vi "Test.vi"   [LabVIEW 2018, in "Scripts.lvlib"]
uses:
  Scripts.lvlib
  <vilib>/addons/_JKI Toolkits/Caraya/classes/Test/Test.lvclass
  tests/Toolkit/Toolkit.lvlib
  <vilib>/Field R&D Services/Labricator/Toolkit/Labricator.lvlib
panel:
  # "Overview: Runs all of tests this project\nRequirements: LabVIEW, Caraya Unit Test Framework \nInstructions: Run this VI.\n\nThis VI runs all of the integration and unit tests."
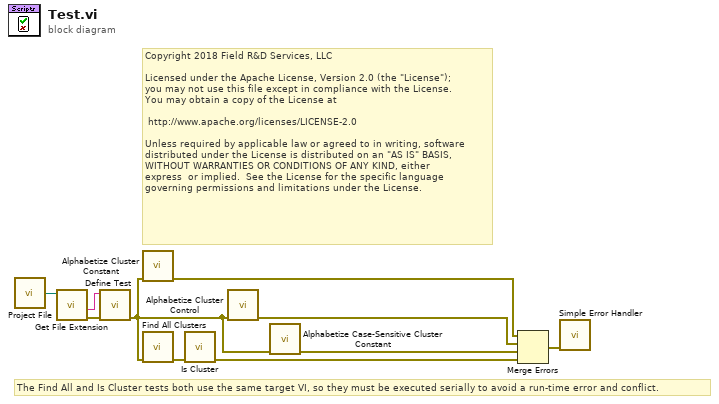
[diagram p0: block diagram]
diagram:
  # "The Find All and Is Cluster tests both use the same target VI, so they must be executed serially to avoid a run-time error and conflict."
  # "Copyright 2018 Field R&D Services, LLC\n\nLicensed under the Apache License, Version 2.0 (the \"License\");\nyou may not use this file except in compliance with the License.\nYou may obtain a copy of the License at\n\n\thttp://www.apache.org/licenses/LICENSE-2.0\n\nUnless required by applicable law or agreed to in writing, software\ndistributed under the License is distributed on an \"AS IS\" BASIS,\nWITHOUT WARRANTIES OR CONDITIONS OF ANY KIND, either \nexpress  or implied.  See the License for the specific language \ngoverning permissions and limitations under the License."
  n1 = call <vilib>:"Project File.vi"() -> ("Project File"=w3:path)
  n2 = call <vilib>:"Get File Extension.vi"("file"=w3) -> ("error out"=w9:errorcluster, "filename without extension"=w10:string)  [unwired: 6 in, 3 out]
  n3 = call <vilib>:"Define Test.vi"("error in (no error)"=w9, "Label (VI Title)"=w10) -> ("error out"=w2:errorcluster)  [unwired: 9 in]
  n4 = call "Alphabetize Cluster Constant.vi"("Error In"=w2) -> ("Error Out"=w8:errorcluster)  [unwired: 10 in]
  n5 = call "Find All Clusters.vi"("Error In"=w2) -> ("Error Out"=w4:errorcluster)  [unwired: 10 in]
  n6 = call "Is Cluster.vi"("Error In"=w4) -> ("Error Out"=w5:errorcluster)  [unwired: 10 in]
  n7 = call "Alphabetize Cluster Control.vi"("Error In"=w2) -> ("Error Out"=w7:errorcluster)  [unwired: 10 in]
  n8 = call "Alphabetize Case-Sensitive Cluster Constant.vi"("Error In"=w2) -> ("Error Out"=w1:errorcluster)  [unwired: 10 in]
  n9 = Merge Errors(w8, w7, w1, w5) -> (w6:errorcluster)
  n10 = call <vilib>:"Simple Error Handler.vi"("error in (no error)"=w6) -> ()  [unwired: 4 in, 5 out]
